vi "Dispose.vi"(0 "reference in":refnum<class "G#Interface.lvclass">, 5 "error in (no error)":errorcluster) -> (14 "reference out":refnum<class "G#Interface.lvclass">, 19 "error out":errorcluster)   [LabVIEW 2020, in "G#Interface.lvclass"]
doc: "Dispose all resources use by the object. This method will call dispose on all aggregated objects and then destroy them."
uses:
  G#Interface.lvclass
  G#Interface.lvclass/G#Interface.ctl
  G#Object/G#Object.lvclass
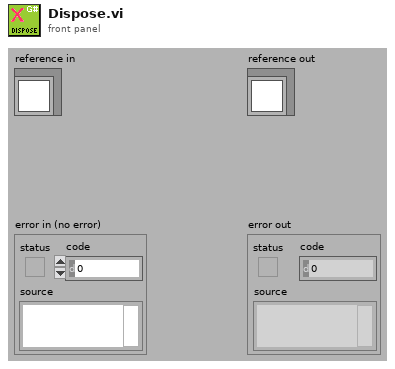
[diagram p1: front panel]
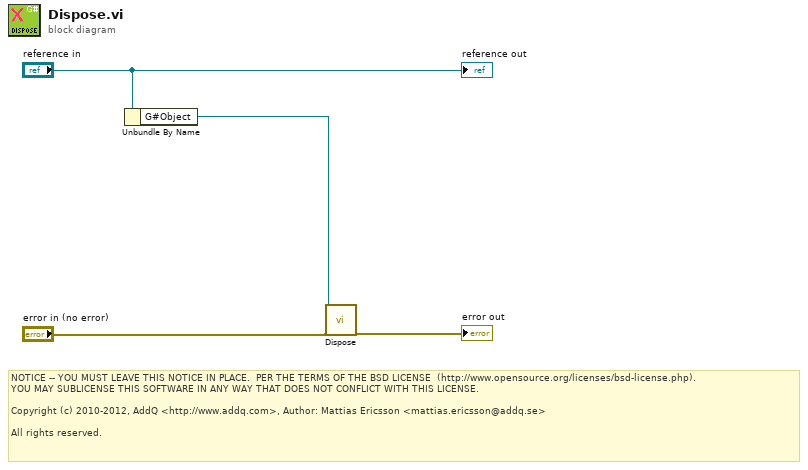
[diagram p0: block diagram]
diagram:
  # "NOTICE -- YOU MUST LEAVE THIS NOTICE IN PLACE.  PER THE TERMS OF THE BSD LICENSE  (http://www.opensource.org/licenses/bsd-license.php).\nYOU MAY SUBLICENSE THIS SOFTWARE IN ANY WAY THAT DOES NOT CONFLICT WITH THIS LICENSE.\n\nCopyright (c) 2010-2012, AddQ <http://www.addq.com>, Author: Mattias Ericsson <mattias.ericsson@addq.se>\n\nAll rights reserved."
  n1 = Unbundle By Name("reference in") -> ("G#Object"=w1:refnum<class "G#Object.lvclass">)
  n2 = call-dynamic "Dispose.vi"("reference in"=w1, "error in (no error)"="error in (no error)") -> ("error out"=→"error out":errorcluster)  [unwired: 16 in, 1 out]
  "reference out" <- "reference in"
